vi "Boiler.vi"() -> ()   [LabVIEW 2015]
uses:
  Controls/Boiler Controls.ctl
  Controls/Boiler Simulation Controls.ctl
  Controls/Boiler Status Indicators.ctl
  Controls/UI Data.ctl
  support/Message Queue/Enqueue Message (Single).vi
  <vilib>/Utility/file.llb/Write Delimited Spreadsheet (string).vi
  <vilib>/Utility/error.llb/Error Cluster From Error Code.vi
  <vilib>/ErrorRing/Error Ring.xnode
  support/Message Queue/Message Queue.lvlib
  support/User Event - Stop/User Event - Stop.lvlib
panel:
  in  "stop":bool
  out "Boiler Status Indicators":T1 {"Time Count" format="%.2g"}
  in  "Boiler Simulation Controls":T2 {"Flame Sensor Value (%)" min=0.0 max=100.0 scale=0.0..100.0}
  in  "Boiler Controls":T3 {"Fuel Valve Position" min=0.0 max=100.0 scale=0.0..100.0 scale format="%.2f"}
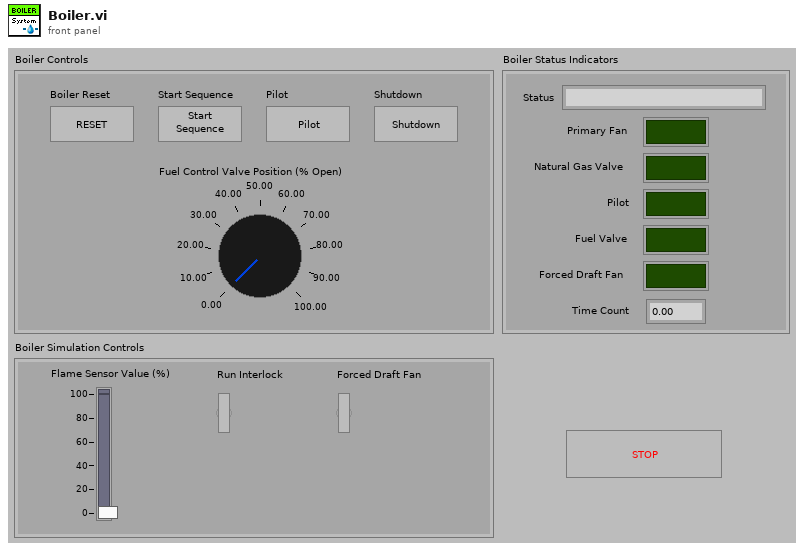
[diagram p1: front panel]
types:
  T1 = typedef "Boiler Status Indicators.ctl" = cluster{"Status":string, "Primary Fan":bool, "Natural Gas Valve":bool, "Pilot":bool, "Fuel Valve":bool, "Forced Draft Fan":bool, "Time Count":dbl}
  T2 = typedef "Boiler Simulation Controls.ctl" = cluster{"Flame Sensor Value (%)":dbl, "Run Interlock":bool, "Forced Draft Fan":bool}
  T3 = typedef "Boiler Controls.ctl" = cluster{"Boiler Reset":bool, "Start Sequence":bool, "Pilot":bool, "Shutdown":bool, "Fuel Valve Position":dbl}
  T4 = typedef "UI Data.ctl" = cluster{"Boolean <Replace Me>":bool, "String <Replace Me>":string, "Numeric <Replace Me>":dbl, "Do Something Ref":refnum<vi>, "Do Something Else Ref":refnum<vi>, "Data Display Ref":refnum<vi>, "Exit Button Ref":refnum<vi>}
  T5 = typedef "Message Queue.lvlib/All Message Queues.ctl" = cluster{"UI":refnum<queue>}
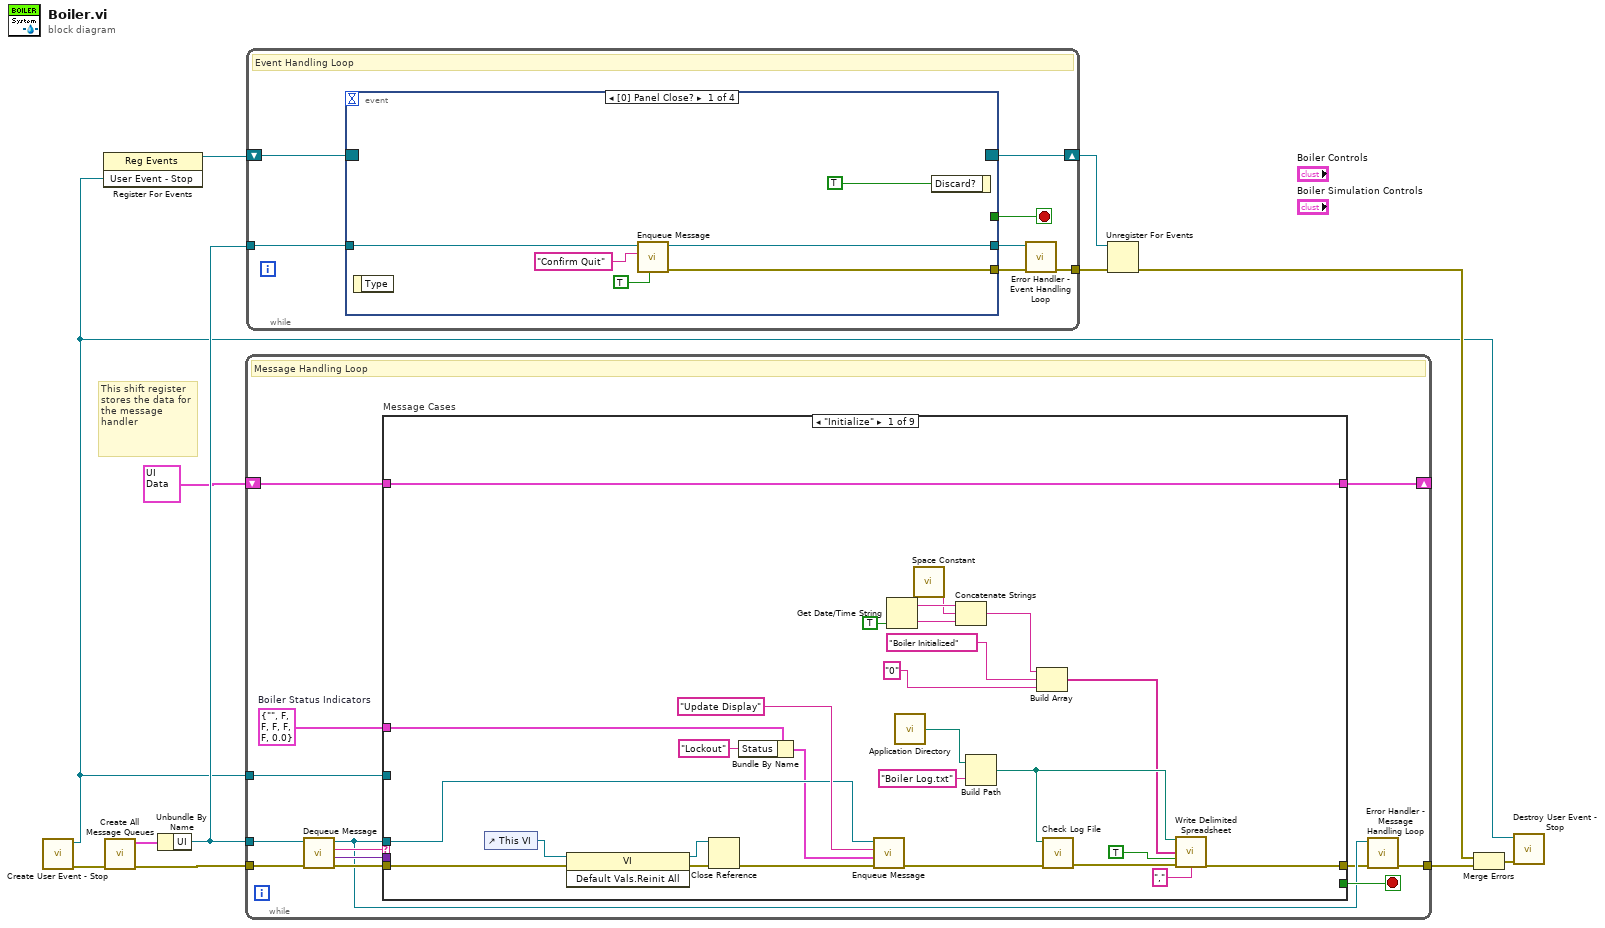
[diagram p0: block diagram]
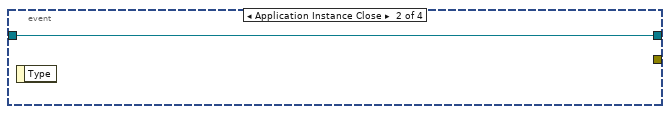
[diagram p2: hidden frame]
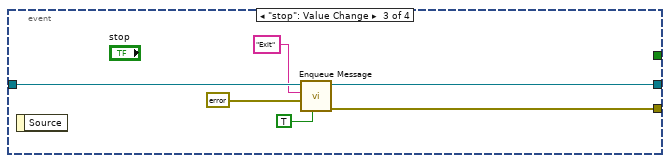
[diagram p3: hidden frame]
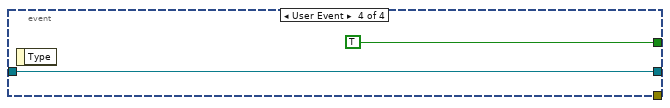
[diagram p4: hidden frame]
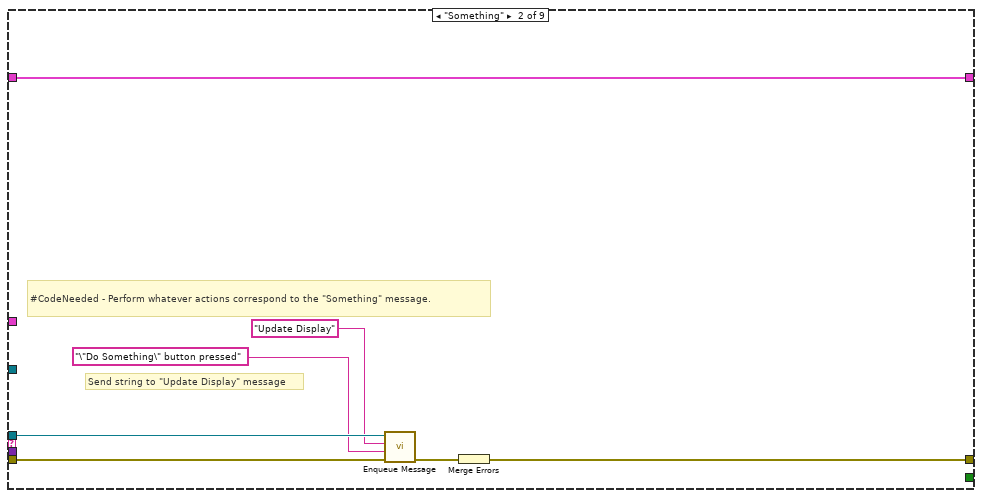
[diagram p5: hidden frame]
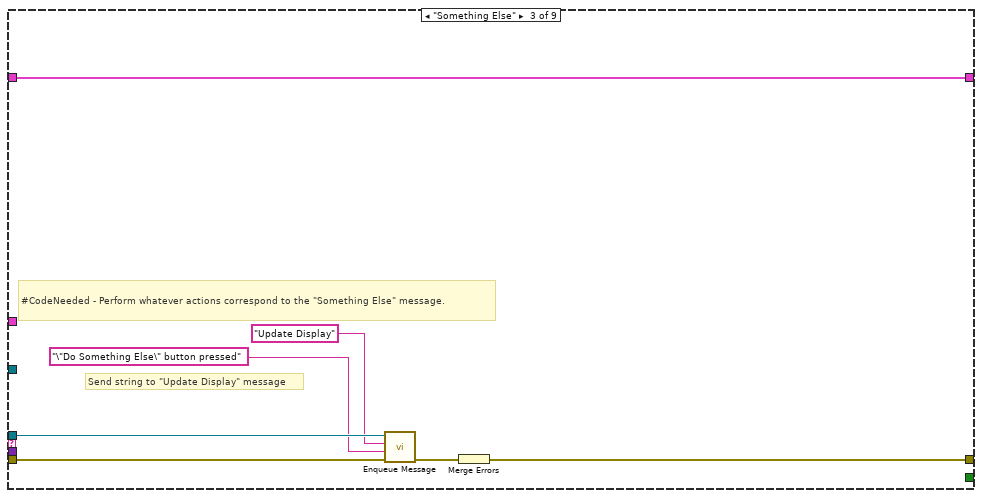
[diagram p6: hidden frame]
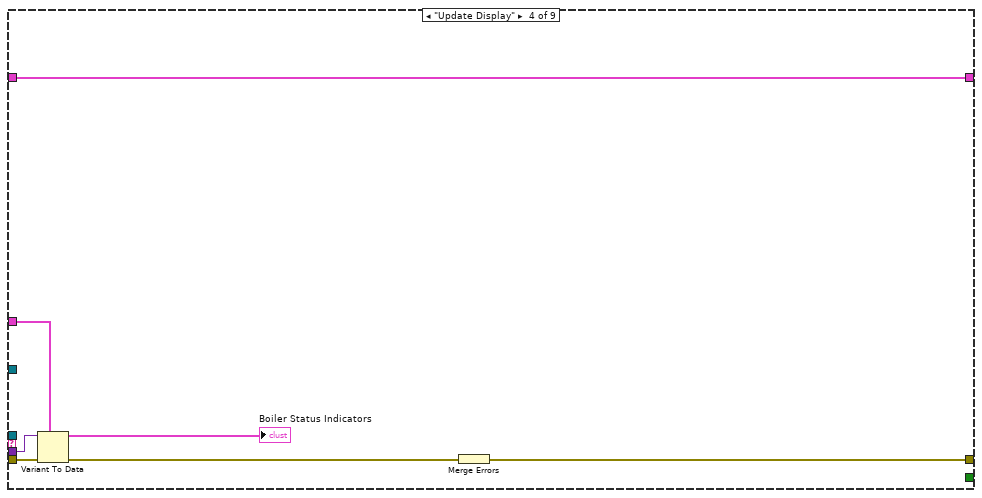
[diagram p7: hidden frame]
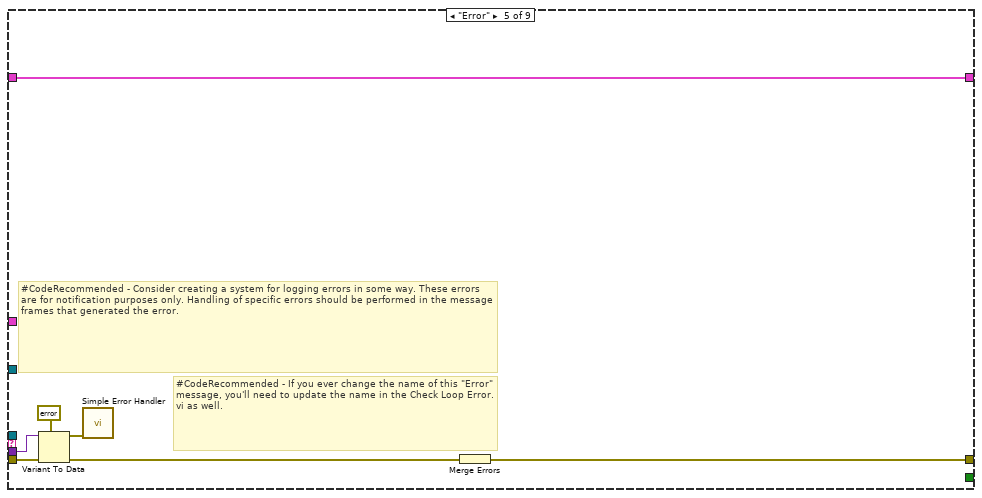
[diagram p8: hidden frame]
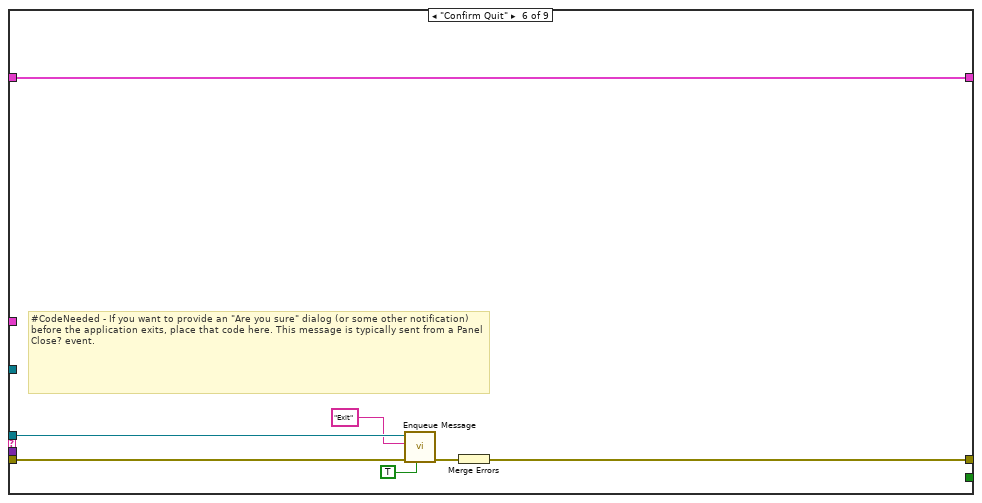
[diagram p9: hidden frame]
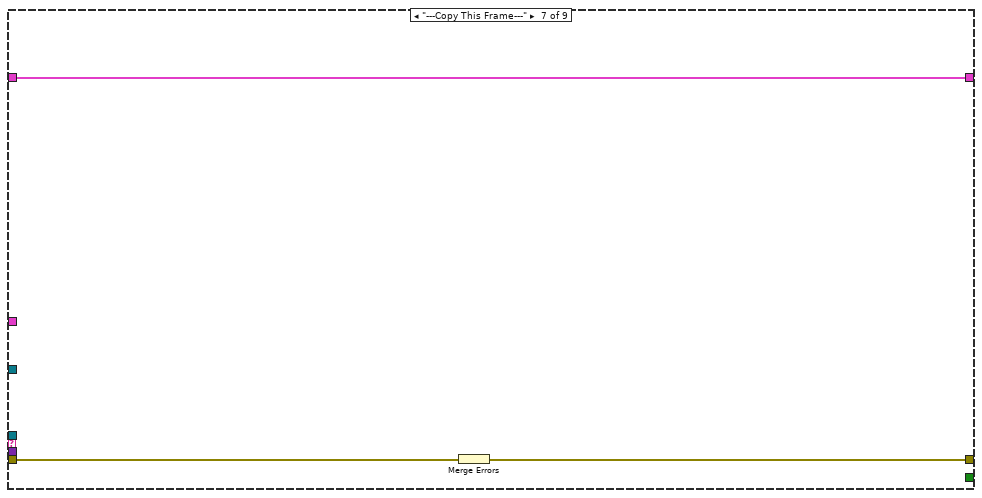
[diagram p10: hidden frame]
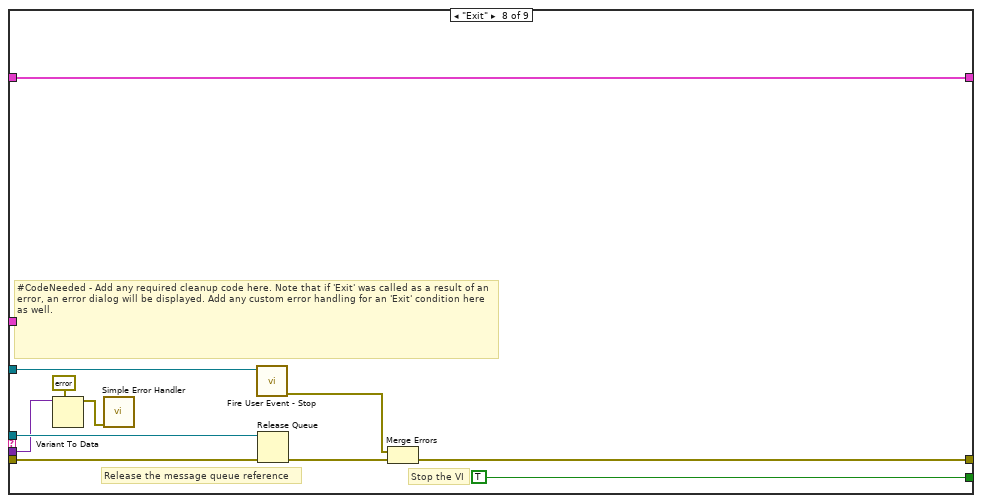
[diagram p11: hidden frame]
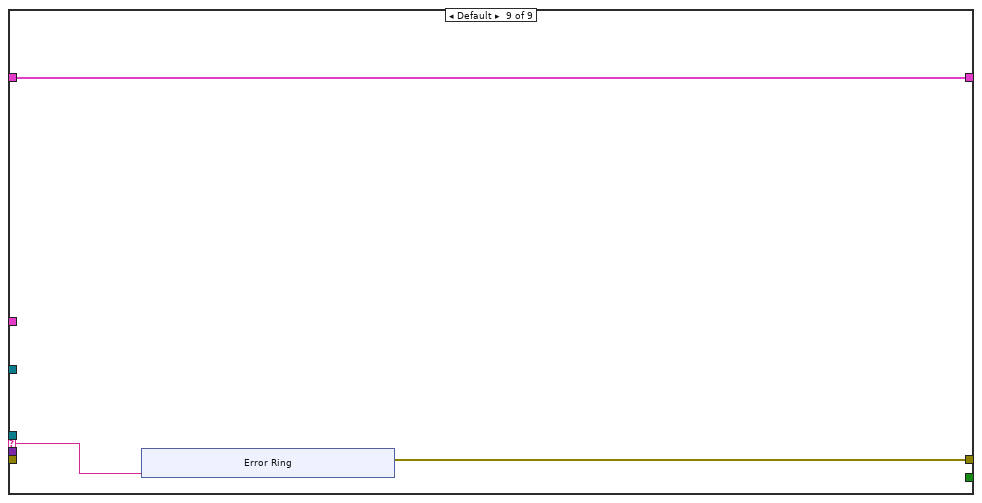
[diagram p12: hidden frame]
diagram:
  # "This shift register stores the data for the message handler"
  n1 = call "Create User Event - Stop.vi"() -> ("error out"=w8:errorcluster, "User Event - Stop"=w1:refnum<user-event>)  [unwired: 10 in]
  n2 = register-events(w1) -> (reference out=w2:refnum<event-registration>)  [unwired: 2 in, 1 out]
  n3 = call "Create All Message Queues.vi"("error in (no error)"=w8) -> ("error out"=w12:errorcluster, "Message Queues out"=w11:T5)  [unwired: 9 in]
  n4 = Unbundle By Name(w11) -> ("UI"=w9:refnum<queue>)
  n5 = while {
    tunnel: w9 -> [w17]
    shift-right: [w24] -> _
    shift-left: T4 {"Boolean <Replace Me>"=FALSE, "String <Replace Me>"="", "Numeric <Replace Me>"=0.0, "Do Something Ref"=refnum, "Do Something Else Ref"=refnum, "Data Display Ref"=refnum, "Exit Button Ref"=refnum} ("Data Cluster") -> [w25]
    tunnel: w1 -> [w22]
    tunnel: w12 -> [w21]
    tunnel: [w15] -> w10
    stop <- w23 stop-if-true
    w13 = T1 {"Status"="", "Primary Fan"=FALSE, "Natural Gas Valve"=FALSE, "Pilot"=FALSE, "Fuel Valve"=FALSE, "Forced Draft Fan"=FALSE, "Time Count"=0.0}  # Boiler Status Indicators
    # "Message Handling Loop"
    n6 = call "Dequeue Message.vi"("error in (no error)"=w21, "Message Queue"=w17) -> ("error out"=w20:errorcluster, "Message Data"=w18:variant, "Message"=w19:string, "dup Message Queue"=w16:refnum<queue>)  [unwired: 6 in]
    n7 = case "Message Cases" shown="\"Initialize\"" w19 {
      selector: w19 -> [_ _ _ _ _ _ _ _ w102]
      tunnel: w16 -> [w49 w55 w62 _ _ w83 _ w101 _]
      tunnel: w20 -> [w45 w57 w64 w71 w80 w87 w90 w94 _]
      tunnel: [w36 w58 w65 w72 w74 w85 w88 w97 w103] -> w14
      tunnel: w25 -> [w51 w59 w66 w73 w79 w86 w89 w100 w104]
      tunnel: [w51 w59 w66 w73 w79 w86 w89 w100 w104] -> w24
      tunnel: [_ _ _ _ _ _ _ TRUE _] -> w23
      tunnel: w18 -> [_ _ _ w70 w78 _ _ w91 _]
      tunnel: w22 -> [_ _ _ _ _ _ _ w96 _]
      tunnel: w13 -> [w48 _ _ w68 _ _ _ _ _]
      frame "Initialize" {
        # "Initialize - All initialization work should take place in this message, since other loops can potentially enqueue messages that execute immediately after this one."
        n8 = control-ref of="This VI"() -> (w44:refnum<vi>)
        n9 = invoke class="VI" method="Default Vals.Reinit All"(reference=w44, error in=w45) -> (reference out=w42:refnum<vi>, error out=w43:errorcluster)  [unwired: 1 in, 1 out]
        n10 = Close Reference(reference=w42, error in (no error)=w43) -> (error out=w41:errorcluster)
        n11 = Bundle By Name(cluster=w48, "Status"="Lockout") -> (w46:T1)
        n12 = call-poly "Enqueue Message.vi"("error in (no error)"=w41, "Message Data"=w46, "Message"="Update Display", "Message Queue"=w49) -> ("error out"=w52:errorcluster)  [unwired: 6 in, 1 out]
        n13 = Get Date/Time String(want seconds? (F)=TRUE) -> (date string=w33:string, time string=w31:string)  [unwired: 2 in]
        n14 = call <vilib>:"Application Directory.vi"() -> ("Application Directory"=w40:path)
        n15 = call <vilib>:"Space Constant.vi"() -> ("String"=w32:string)
        n16 = Concatenate Strings(w33, w32, w31) -> (w30:string)
        n17 = Build Path(base path=w40, name or relative path="Boiler Log.txt") -> (appended path=w35:path)
        n18 = Build Array(w30, "Boiler Initialized", "0") -> (w28:string[])
        n19 = call "Check Log File.vi"("Error In"=w52, "Log File Path"=w35) -> ("Error Out"=w38:errorcluster)  [unwired: 9 in]
        n20 = call-poly <vilib>:"Write Delimited Spreadsheet.vi"("file path (dialog if empty)"=w35, "1D data"=w28, "append to file? (F)"=TRUE, "error in (no error)"=w38, "delimiter (\\t)"="," ("delimiter (\\t)")) -> ("error out"=w36:errorcluster)  [unwired: 9 in, 1 out]
      }
      frame "Something" {
        # "Send string to \"Update Display\" message"
        # "#CodeNeeded - Perform whatever actions correspond to the \"Something\" message."
        # "Something - Replace this message with functionality for your own application."
        n21 = call-poly "Enqueue Message.vi"("error in (no error)"=w57, "Message Data"="\"Do Something\" button pressed" ("\"Do Something\" button pressed"), "Message"="Update Display", "Message Queue"=w55) -> ("error out"=w56:errorcluster)  [unwired: 6 in, 1 out]
        n22 = Merge Errors(w56) -> (w58:errorcluster)
      }
      frame "Something Else" {
        # "Send string to \"Update Display\" message"
        # "#CodeNeeded - Perform whatever actions correspond to the \"Something Else\" message."
        # "Something Else - Replace this message with functionality for your own application."
        n23 = call-poly "Enqueue Message.vi"("error in (no error)"=w64, "Message Data"="\"Do Something Else\" button pressed" ("\"Do Something Else\" button pressed"), "Message"="Update Display", "Message Queue"=w62) -> ("error out"=w63:errorcluster)  [unwired: 6 in, 1 out]
        n24 = Merge Errors(w63) -> (w65:errorcluster)
      }
      frame "Update Display" {
        # "Update Display - Convert the message data to a string to display in the Data Display indicator."
        n25 = Variant To Data(error in=w71, type=w68, Variant=w70) -> (data=→"Boiler Status Indicators":T1, error out=w69:errorcluster)
        n26 = Merge Errors(w69) -> (w72:errorcluster)
      }
      frame "Error" {
        # "#CodeRecommended - If you ever change the name of this \"Error\" message, you'll need to update the name in the Check Loop Error.vi as well."
        # "#CodeRecommended - Consider creating a system for logging errors in some way. These errors are for notification purposes only. Handling of specific errors should be performed in the message frames that generated the error."
        # "Error - Display an error dialog. This message is sent by the \"Error Handler\" VIs at the end of other loops in this application."
        n27 = Variant To Data(error in=w80, type=errorcluster {"status"=FALSE, "code"=0, "source"=""} ("error constant"), Variant=w78) -> (data=w76:errorcluster, error out=w75:errorcluster)
        n28 = call <vilib>:"Simple Error Handler.vi"("error in (no error)"=w76) -> ()  [unwired: 4 in, 5 out]
        n29 = Merge Errors(w75) -> (w74:errorcluster)
      }
      frame "Confirm Quit" {
        # "#CodeNeeded - If you want to provide an \"Are you sure\" dialog (or some other notification) before the application exits, place that code here. This message is typically sent from a Panel Close? event."
        # "Confirm Quit - Message that can confirm whether or not the user wants to exit the application."
        n30 = call-poly "Enqueue Message.vi"("Priority Message? (F)"=TRUE, "error in (no error)"=w87, "Message"="Exit", "Message Queue"=w83) -> ("error out"=w84:errorcluster)  [unwired: 6 in, 1 out]
        n31 = Merge Errors(w84) -> (w85:errorcluster)
      }
      frame "---Copy This Frame---" {
        # "Duplicate this frame when creating new messages.  Change this comment in the duplicated frame to describe this message."
        n32 = Merge Errors(w90) -> (w88:errorcluster)
      }
      frame "Exit" {
        # "Stop the VI"
        # "Release the message queue reference"
        # "#CodeNeeded - Add any required cleanup code here. Note that if 'Exit' was called as a result of an error, an error dialog will be displayed. Add any custom error handling for an 'Exit' condition here as well."
        # "Exit - Exit the application."
        n33 = Variant To Data(type=errorcluster {"status"=FALSE, "code"=0, "source"=""} ("error constant"), Variant=w91) -> (data=w92:errorcluster)  [unwired: 1 in, 1 out]
        n34 = call <vilib>:"Simple Error Handler.vi"("error in (no error)"=w92) -> ()  [unwired: 4 in, 5 out]
        n35 = call "Fire User Event - Stop.vi"("User Event - Stop"=w96) -> ("error out"=w95:errorcluster)  [unwired: 10 in]
        n36 = Release Queue(queue=w101, error in (no error)=w94) -> (error out=w98:errorcluster)  [unwired: 1 in, 2 out]
        n37 = Merge Errors(w95, w98) -> (w97:errorcluster)
      }
      frame Default {
        # "'Default' case only runs if there is a message that isn't defined in any of the other cases.  Output a programming error."
        n38 = xnode "Error Ring"("parameter 0"=w102) -> ("error out"=w103:errorcluster)
      }
    }
    n39 = call "Error Handler - Message Handling Loop.vi"("error in (no error)"=w14, "Message Queue"=w16) -> ("dup error in"=w15:errorcluster)  [unwired: 8 in, 1 out]
  }
  n40 = while {
    tunnel: w9 -> [w118]
    shift-right: [w116] -> w5
    shift-left: w2 -> [w117]
    tunnel: [w112] -> w3
    stop <- w114 stop-if-true
    # "Event Handling Loop"
    n41 = event shown="[0] Panel Close?" {
      selector: w117 -> [_ _ _ _]
      dyn-events: [_ _ _ _] -> w116
      timeout: _ -> [_ _ _ _]
      tunnel: [_ _ _ TRUE ("Discard?")] -> w114
      tunnel: w118 -> [w123 w125 w131 w133]
      tunnel: [w122 _ w130 _] -> w115
      tunnel: [w121 w125 w129 w133] -> w113
      event Panel Close? {
        n42 = event-data() -> ()  [unwired: 1 in, 1 out]
        n43 = call-poly "Enqueue Message.vi"("Priority Message? (F)"=TRUE, "Message"="Confirm Quit", "Message Queue"=w123) -> ("error out"=w122:errorcluster, "dup Message Queue"=w121:refnum<queue>)  [unwired: 7 in]
        n44 = event-data("Discard?"=TRUE) -> ()  [unwired: 1 in, 1 out]
      }
      event Application Instance Close {
        n45 = event-data() -> ()  [unwired: 1 in, 1 out]
      }
      event "stop": Value Change {
        n46 = event-data() -> ()  [unwired: 1 in, 1 out]
        n47 = call-poly "Enqueue Message.vi"("Priority Message? (F)"=TRUE, "Message Data"=errorcluster {"status"=FALSE, "code"=0, "source"=""} ("error out"), "Message"="Exit", "Message Queue"=w131) -> ("error out"=w130:errorcluster, "dup Message Queue"=w129:refnum<queue>)  [unwired: 6 in]
      }
      event User Event {
        n48 = event-data() -> ()  [unwired: 1 in, 1 out]
      }
    }
    n49 = call "Error Handler - Event Handling Loop.vi"("error in (no error)"=w115, "Message Queue"=w113) -> ("dup error in"=w112:errorcluster)  [unwired: 8 in, 1 out]
  }
  n50 = Unregister For Events(event registration refnum=w5, error in=w3) -> (error out=w6:errorcluster)
  n51 = Merge Errors(w6, w10) -> (w7:errorcluster)
  n52 = call "Destroy User Event - Stop.vi"("error in (no error)"=w7, "User Event - Stop"=w1) -> ()  [unwired: 9 in, 1 out]
